vi "c_Handle subWorker Error.vi"() -> (1 "Case Label":T1)   [LabVIEW 2017, in "Method 1.lvlib" / "Head Worker.lvclass"]
doc: "This VI contains a string constant containing the name of a MHL case of the Worker that owns this VI."
uses:
  Head Worker.lvclass
  <vilib>/addons/_Workers/Library/Case Label.ctl
  <vilib>/addons/_Workers/Library/Workers.lvlib
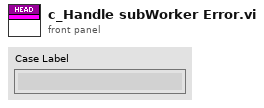
[diagram p1: front panel]
types:
  T1 = typedef "Workers.lvlib/Case Label.ctl" = string
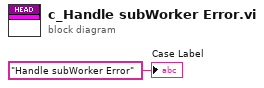
[diagram p0: block diagram]
diagram:
  "Case Label" <- T1 "Handle subWorker Error" ("Case Label")
